vi "总磷氨氮量程写入.vi"(7 "量程切换阈值":cluster{"阈值":dbl, "标液浓度":dbl}, 8 "error in (no error)":errorcluster caption="错误输入（无错误）", 9 "量程":enum16{"低量程", "高量程"}(ring), 10 "测量模式":enum16{"水样测量", "空白核查", "标样核查", "盲样测试", "加标回收"}(ring), 11 "测量参数":enum16{"氨氮", "总磷"}(ring)) -> (0 "error out":errorcluster caption="错误输出")   [LabVIEW 2016, in "氨氮总磷.lvlib"]
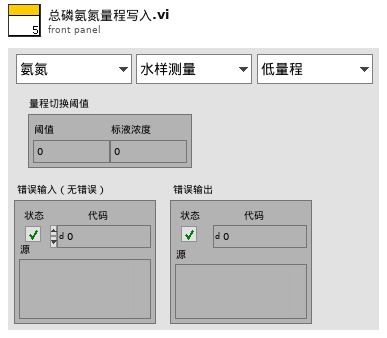
[diagram p1: front panel]
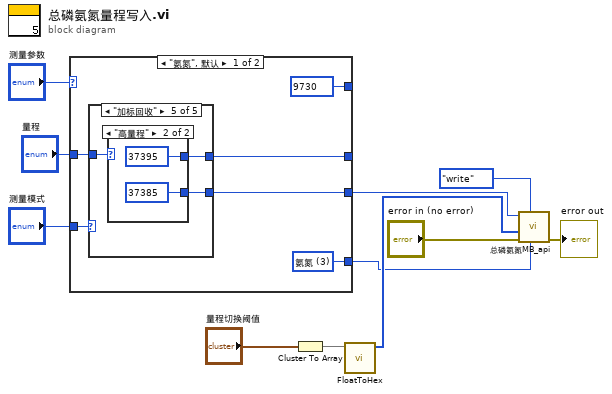
[diagram p0: block diagram]
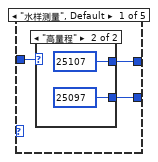
[diagram p2: hidden frame]
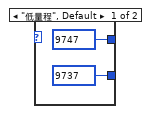
[diagram p3: hidden frame]
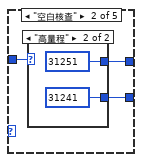
[diagram p4: hidden frame]
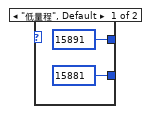
[diagram p5: hidden frame]
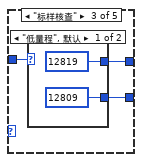
[diagram p6: hidden frame]
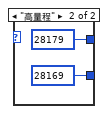
[diagram p7: hidden frame]
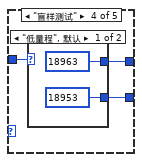
[diagram p8: hidden frame]
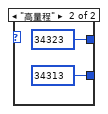
[diagram p9: hidden frame]
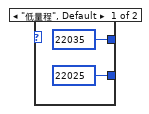
[diagram p10: hidden frame]
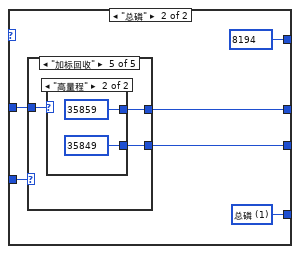
[diagram p11: hidden frame]
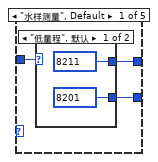
[diagram p12: hidden frame]
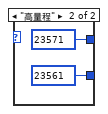
[diagram p13: hidden frame]
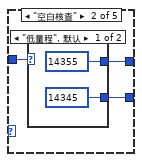
[diagram p14: hidden frame]
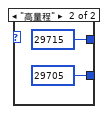
[diagram p15: hidden frame]
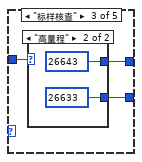
[diagram p16: hidden frame]
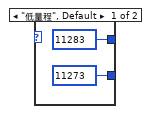
[diagram p17: hidden frame]
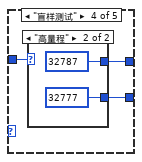
[diagram p18: hidden frame]
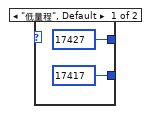
[diagram p19: hidden frame]
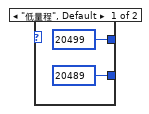
[diagram p20: hidden frame]
diagram:
  n1 = case shown="\"氨氮\", 默认" "测量参数" {
    tunnel: "测量模式" -> [w17 w58]
    tunnel: "量程" -> [w16 w57]
    tunnel: [w15 w56] -> w1
    tunnel: [w14 w55] -> _
    tunnel: [w13 w54] -> w8
    tunnel: [u16 9730 ("starting address") u16 8194 ("starting address")] -> _
    frame "氨氮", Default {
      w15 = u16 3 items=["总磷"=1, "氨氮"=3] ("站号")
      n2 = case shown="\"加标回收\"" w17 {
        tunnel: w16 -> [w20 w27 w34 w41 w48]
        tunnel: [w19 w26 w33 w40 w47] -> w14
        tunnel: [w18 w25 w32 w39 w46] -> w13
        frame "水样测量", Default {
          n3 = case shown="\"高量程\"" w20 {
            tunnel: [u16 9747 ("starting address") u16 25107 ("starting address")] -> w19
            tunnel: [u16 9737 ("starting address") u16 25097 ("starting address")] -> w18
            frame "低量程", Default {
            }
            frame "高量程" {
            }
          }
        }
        frame "空白核查" {
          n4 = case shown="\"高量程\"" w27 {
            tunnel: [u16 15891 ("starting address") u16 31251 ("starting address")] -> w26
            tunnel: [u16 15881 ("starting address") u16 31241 ("starting address")] -> w25
            frame "低量程", Default {
            }
            frame "高量程" {
            }
          }
        }
        frame "标样核查" {
          n5 = case shown="\"低量程\", 默认" w34 {
            tunnel: [u16 12819 ("starting address") u16 28179 ("starting address")] -> w33
            tunnel: [u16 12809 ("starting address") u16 28169 ("starting address")] -> w32
            frame "低量程", Default {
            }
            frame "高量程" {
            }
          }
        }
        frame "盲样测试" {
          n6 = case shown="\"低量程\", 默认" w41 {
            tunnel: [u16 18963 ("starting address") u16 34323 ("starting address")] -> w40
            tunnel: [u16 18953 ("starting address") u16 34313 ("starting address")] -> w39
            frame "低量程", Default {
            }
            frame "高量程" {
            }
          }
        }
        frame "加标回收" {
          n7 = case shown="\"高量程\"" w48 {
            tunnel: [u16 22035 ("starting address") u16 37395 ("starting address")] -> w47
            tunnel: [u16 22025 ("starting address") u16 37385 ("starting address")] -> w46
            frame "低量程", Default {
            }
            frame "高量程" {
            }
          }
        }
      }
    }
    frame "总磷" {
      w56 = u16 1 items=["总磷"=1, "氨氮"=3] ("站号")
      n8 = case shown="\"加标回收\"" w58 {
        tunnel: w57 -> [w61 w68 w75 w82 w89]
        tunnel: [w60 w67 w74 w81 w88] -> w55
        tunnel: [w59 w66 w73 w80 w87] -> w54
        frame "水样测量", Default {
          n9 = case shown="\"低量程\", 默认" w61 {
            tunnel: [u16 8211 ("starting address") u16 23571 ("starting address")] -> w60
            tunnel: [u16 8201 ("starting address") u16 23561 ("starting address")] -> w59
            frame "低量程", Default {
            }
            frame "高量程" {
            }
          }
        }
        frame "空白核查" {
          n10 = case shown="\"低量程\", 默认" w68 {
            tunnel: [u16 14355 ("starting address") u16 29715 ("starting address")] -> w67
            tunnel: [u16 14345 ("starting address") u16 29705 ("starting address")] -> w66
            frame "低量程", Default {
            }
            frame "高量程" {
            }
          }
        }
        frame "标样核查" {
          n11 = case shown="\"高量程\"" w75 {
            tunnel: [u16 11283 ("starting address") u16 26643 ("starting address")] -> w74
            tunnel: [u16 11273 ("starting address") u16 26633 ("starting address")] -> w73
            frame "低量程", Default {
            }
            frame "高量程" {
            }
          }
        }
        frame "盲样测试" {
          n12 = case shown="\"高量程\"" w82 {
            tunnel: [u16 17427 ("starting address") u16 32787 ("starting address")] -> w81
            tunnel: [u16 17417 ("starting address") u16 32777 ("starting address")] -> w80
            frame "低量程", Default {
            }
            frame "高量程" {
            }
          }
        }
        frame "加标回收" {
          n13 = case shown="\"高量程\"" w89 {
            tunnel: [u16 20499 ("starting address") u16 35859 ("starting address")] -> w88
            tunnel: [u16 20489 ("starting address") u16 35849 ("starting address")] -> w87
            frame "低量程", Default {
            }
            frame "高量程" {
            }
          }
        }
      }
    }
  }
  n14 = Cluster To Array(cluster="量程切换阈值") -> (array=w4:dbl[])
  n15 = call "FloatToHex.vi"("浮点数"=w4) -> ("DCBA整形输出"=w3:u16[])  [unwired: 10 in]
  n16 = call "总磷氨氮MB_api.vi"("Slave ID"=w1, "STEP"=enum16{"open", "read", "write", "close"}."write", "Error in"="error in (no error)", "values"=w3, "starting address"=w8) -> ("error out"=→"error out":errorcluster)  [unwired: 3 in, 3 out]
